vi "Write Fetch Relative To.vi"(8 "error in (no error)":errorcluster, 10 "Fetch Relative To":i32(ring)=477 items=["Start"=482, "Trigger"=483, "Pretrigger"=477, "Now"=481, "Read Pointer"=388], 11 "Ni-Scope Digitizer in":refnum<class "Ni-Scope Digitizer.lvclass">) -> (0 "error out":errorcluster, 3 "Ni-Scope Digitizer out":refnum<class "Ni-Scope Digitizer.lvclass">)   [LabVIEW 2016, in "Ni-Scope Digitizer.lvclass"]
uses:
  Ni-Scope Digitizer.lvclass
  Ni-Scope Digitizer.lvclass/Ni-Scope Digitizer.ctl
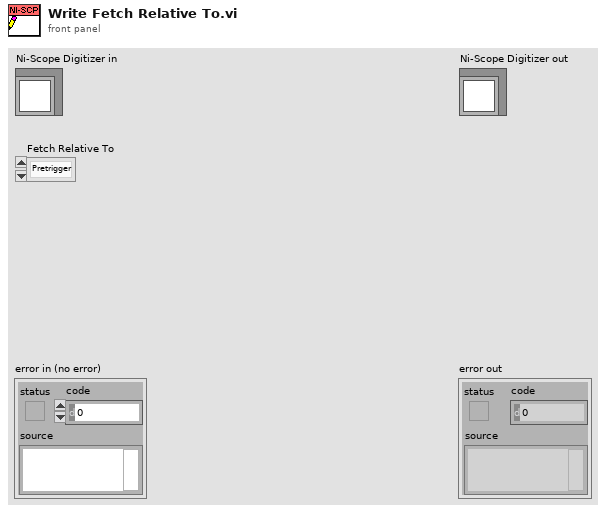
[diagram p1: front panel]
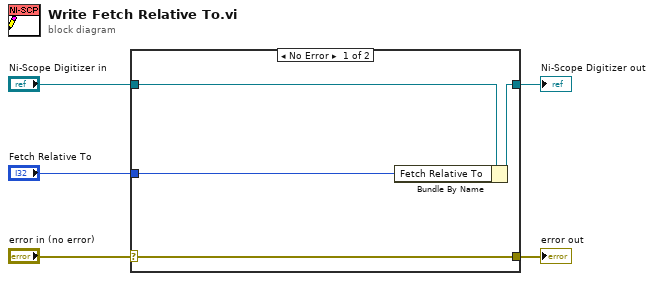
[diagram p0: block diagram]
diagram:
  n1 = case shown="No Error" "error in (no error)" {
    selector: "error in (no error)" -> [w9 w10]
    tunnel: [w9 w10] -> w4
    tunnel: [w7 w11] -> w2
    tunnel: "Ni-Scope Digitizer in" -> [w8 w11]
    tunnel: "Fetch Relative To" -> [w6 _]
    frame No Error {
      n2 = Bundle By Name(cluster=w8, "Fetch Relative To"=w6) -> (w7:refnum<class "Ni-Scope Digitizer.lvclass">)
    }
    frame Error {
    }
  }
  "error out" <- w4
  "Ni-Scope Digitizer out" <- w2
